vi "OADateToTimeStamp.vi"(1 "OADate":dbl=86400.0 format="%#_13g") -> (0 "UTC Time Stamp":timestamp)   [LabVIEW 2021]
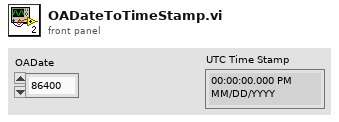
[diagram p1: front panel]
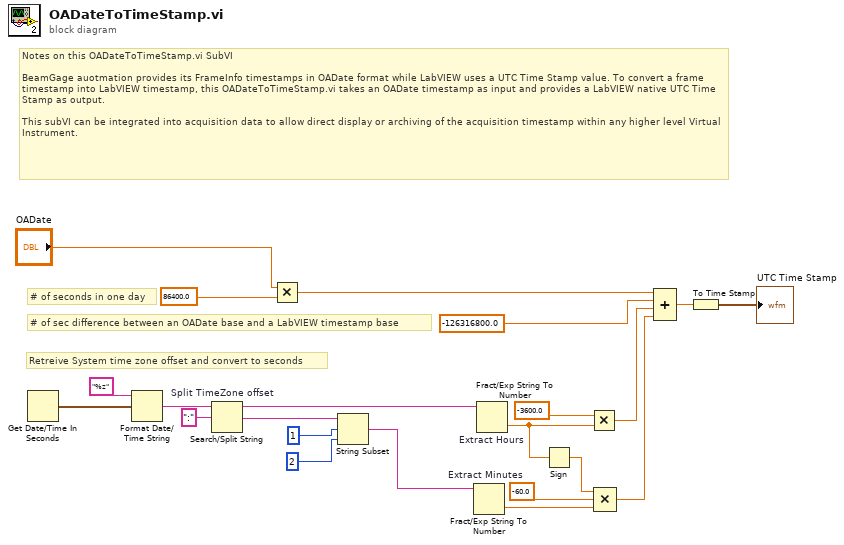
[diagram p0: block diagram]
diagram:
  # "Notes on this OADateToTimeStamp.vi SubVI\n\nBeamGage auotmation provides its FrameInfo timestamps in OADate format while LabVIEW uses a UTC Time Stamp value. To convert a frame timestamp into LabVIEW timestamp, this OADateToTimeStamp.vi takes an OADate timestamp as input and provides a LabVIEW native UTC Time Stamp as output.\n\nThis subVI can be integrated into acquisition data to allow direct display or archiving of the acquisition timestamp within any higher level Virtual Instrument."
  # "Retreive System time zone offset and convert to seconds"
  # "# of seconds in one day"
  # "# of sec difference between an OADate base and a LabVIEW timestamp base"
  n1 = Get Date/Time In Seconds() -> (seconds since 1Jan1904=w11:timestamp)
  n2 = Format Date/Time String(time format string (%c)="%z", seconds (now)=w11) -> (date/time string=w9:string)  [unwired: 1 in]
  n3 = Search/Split String "Split TimeZone offset"(string=w9, search string/char (-)=":") -> (substring before match=w21:string, match + rest of string=w1:string)  [unwired: 1 in, 1 out]
  n4 = Multiply(x="OADate", y=86400.0) -> (x*y=w19:dbl)
  n5 = String Subset(string=w1, offset (0)=1, length (rest)=2) -> (substring=w16:string)
  n6 = Fract/Exp String To Number "Extract Minutes"(string=w16) -> (number=w5:dbl)  [unwired: 3 in, 1 out]
  n7 = Fract/Exp String To Number "Extract Hours"(string=w21) -> (number=w15:dbl)  [unwired: 3 in, 1 out]
  n8 = Sign(1:w15) -> (0:w3:dbl)
  n9 = Multiply(x=-3600.0, y=w15) -> (x*y=w17:dbl)
  n10 = Compound Arithmetic op=MULTIPLY(w3, -60.0 ("x"), w5) -> (w14:dbl)
  n11 = Compound Arithmetic op=ADD(w19, -126316800.0 ("y"), w17, w14) -> (w20:dbl)
  n12 = To Time Stamp(1:w20) -> (0:→"UTC Time Stamp":timestamp)
